vi "Duplicate Stream ID Error.vi"(7 "vi name":string, 8 "error in (no error)":errorcluster, 10 "stream id":u16, 11 "PXImc Transceiver in":refnum<class "DSF PXImc Transceiver.lvclass">=refnum) -> (0 "error out":errorcluster, 3 "PXImc Transceiver out":refnum<class "DSF PXImc Transceiver.lvclass">)   [LabVIEW 2017, in "DSF Core.lvlib" / "DSF PXImc Transceiver.lvclass"]
uses:
  DSF PXImc Transceiver.lvclass
  Errors.ctl
  DSF PXImc Transceiver.lvclass/DSF PXImc Transceiver.ctl
  <vilib>/NI/Memory Manager/VIs/Write Numeric Scalar to Source (Base10 U16).vi
  <vilib>/NI/Memory Manager/Static Errors.lvlib
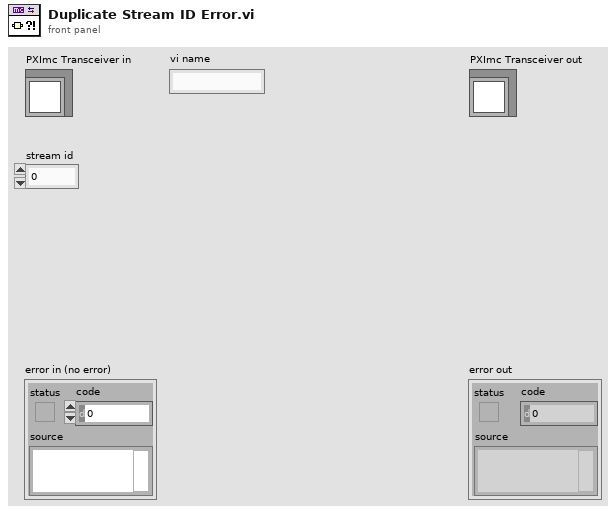
[diagram p1: front panel]
types:
  T1 = typedef "DSF Core.lvlib/DSF PXImc Transceiver.lvclass/Errors.ctl" = enum8{"Bad Setting", "Duplicate Stream ID"}
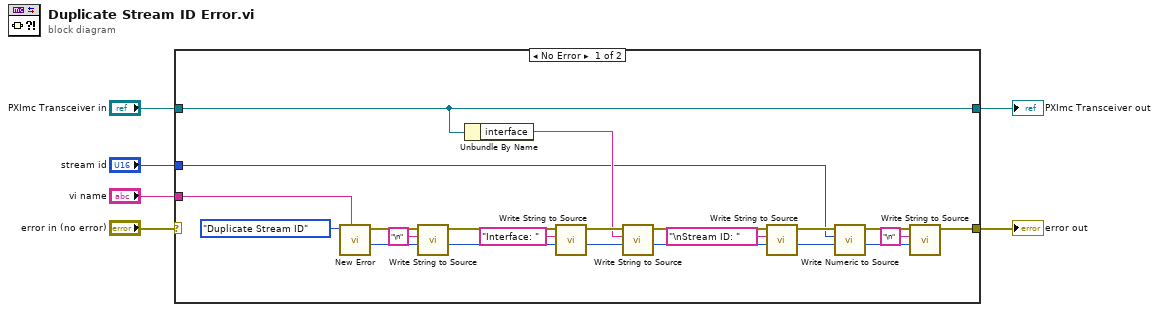
[diagram p0: block diagram]
diagram:
  n1 = case shown="No Error" "error in (no error)" {
    selector: "error in (no error)" -> [_ w30]
    tunnel: [w19 w30] -> w5
    tunnel: [w17 w29] -> w3
    tunnel: "PXImc Transceiver in" -> [w17 w29]
    tunnel: "vi name" -> [w27 _]
    tunnel: "stream id" -> [w7 _]
    frame No Error {
      n2 = call "New Error.vi"("vi name"=w27, "error"=Errors."Duplicate Stream ID") -> ("initial offset"=w18:i32, "error"=w26:errorcluster)  [unwired: 8 in]
      n3 = call <vilib>:"Write String to Source.vi"("offset"=w18, "string"="\n", "error in"=w26) -> ("new offset"=w24:i32, "error out"=w23:errorcluster)  [unwired: 7 in]
      n4 = Unbundle By Name(w17) -> ("interface"=w12:tag)
      n5 = call <vilib>:"Write String to Source.vi"("offset"=w24, "string"="Interface: ", "error in"=w23) -> ("new offset"=w15:i32, "error out"=w16:errorcluster)  [unwired: 7 in]
      n6 = call <vilib>:"Write String to Source.vi"("offset"=w15, "string"=w12, "error in"=w16) -> ("new offset"=w13:i32, "error out"=w14:errorcluster)  [unwired: 7 in]
      n7 = call <vilib>:"Write String to Source.vi"("offset"=w13, "string"="\nStream ID: ", "error in"=w14) -> ("new offset"=w10:i32, "error out"=w11:errorcluster)  [unwired: 7 in]
      n8 = call-poly <vilib>:"Write Numeric to Source.vi"("offset"=w10, "value"=w7, "error in"=w11) -> ("new offset"=w8:i32, "error out"=w9:errorcluster)  [unwired: 7 in]
      n9 = call <vilib>:"Write String to Source.vi"("offset"=w8, "string"="\n", "error in"=w9) -> ("error out"=w19:errorcluster)  [unwired: 7 in, 1 out]
    }
    frame Error {
    }
  }
  "error out" <- w5
  "PXImc Transceiver out" <- w3
